vi "Calculator.vi"() -> ()   [LabVIEW 2014]
uses:
  Calc_States.ctl
panel:
  in  "stop":bool
  out "Operator_In?":bool
  out "Result":dbl
  out "Operator":string
  out "Operand_2":dbl
  out "Operand_1":dbl
  in  ".":bool caption="1 18"
  out "Numeric Indicator":dbl format="%#.13g"
  in  "=":bool caption="1 17"
  in  "%":bool caption="1 16"
  in  "Clr":bool caption="1 15"
  in  "+":bool caption="1 14"
  in  "0":bool caption="1 13"
  in  "/":bool caption="1 12"
  in  "*":bool caption="1 11"
  in  "-":bool caption="1 10"
  in  "9":bool caption="1 9"
  in  "8":bool caption="1 8"
  in  "7":bool
  in  "6":bool caption="1 6"
  in  "5":bool caption="1 5"
  in  "4":bool caption="1 4"
  in  "3":bool caption="1 3"
  in  "2":bool caption="1 2"
  in  "1":bool
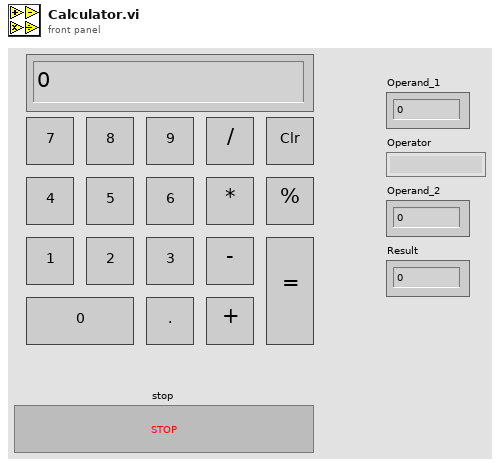
[diagram p1: front panel]
types:
  T1 = typedef "Calc_States.ctl" = cluster{"Calculator State":string, "Key Value":i16}
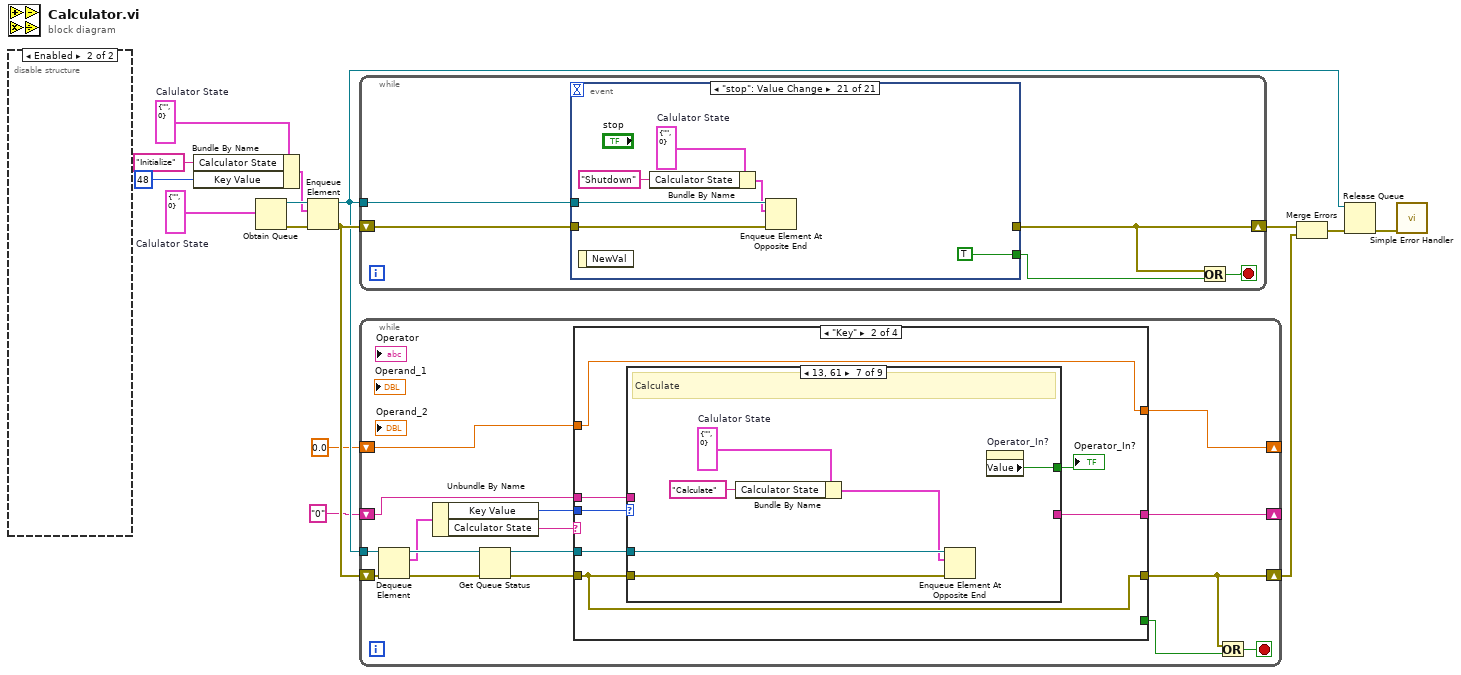
[diagram p0: block diagram]
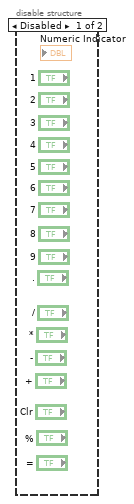
[diagram p2: hidden frame]
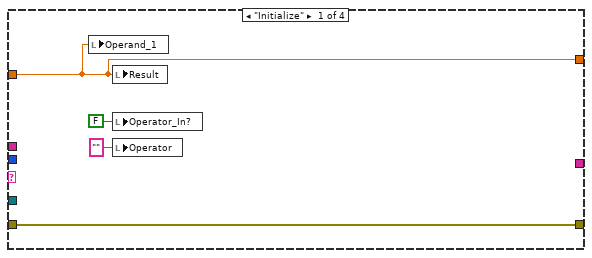
[diagram p3: hidden frame]
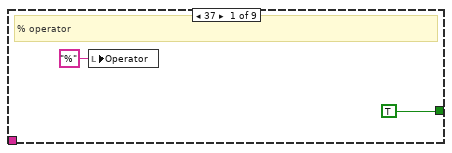
[diagram p4: hidden frame]
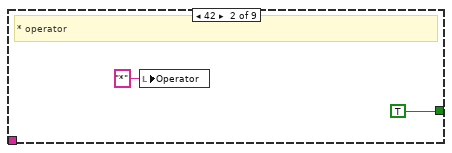
[diagram p5: hidden frame]
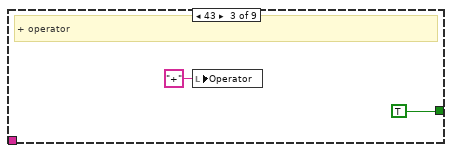
[diagram p6: hidden frame]
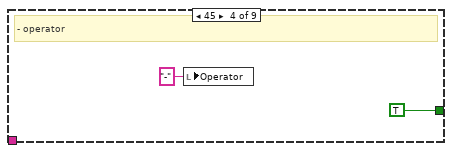
[diagram p7: hidden frame]
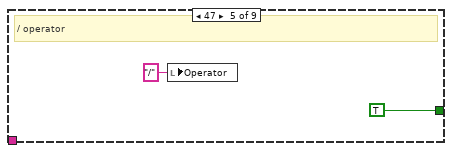
[diagram p8: hidden frame]
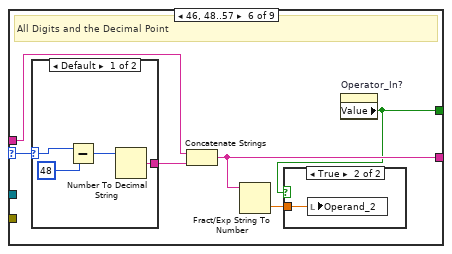
[diagram p9: hidden frame]
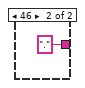
[diagram p10: hidden frame]
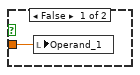
[diagram p11: hidden frame]
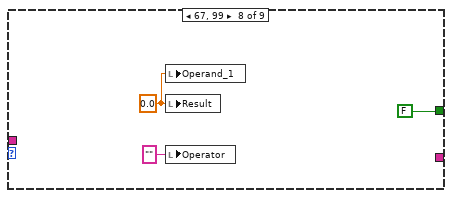
[diagram p12: hidden frame]
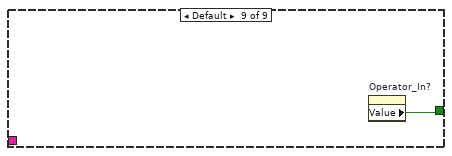
[diagram p13: hidden frame]
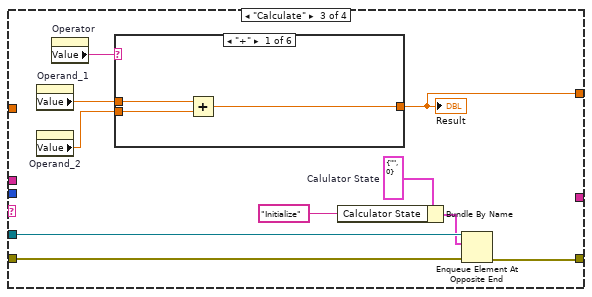
[diagram p14: hidden frame]
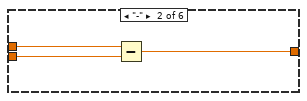
[diagram p15: hidden frame]
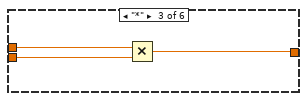
[diagram p16: hidden frame]
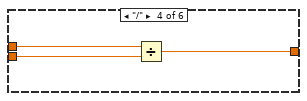
[diagram p17: hidden frame]
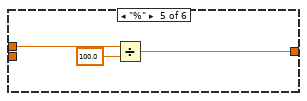
[diagram p18: hidden frame]
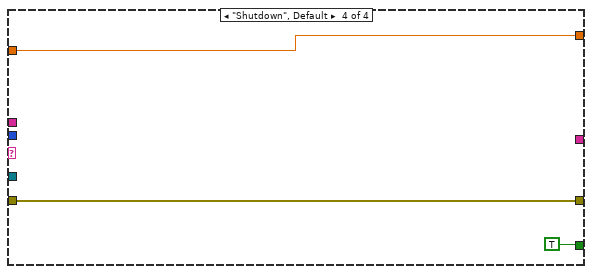
[diagram p20: hidden frame]
diagram:
  w3 = T1 {"Calculator State"="", "Key Value"=0}  # Calulator State
  w8 = T1 {"Calculator State"="", "Key Value"=0}  # Calulator State
  n1 = disable-structure shown="Enabled" {
    frame Disabled {
    }
    frame Enabled {
    }
  }
  n2 = Bundle By Name(cluster=w8, "Calculator State"="Initialize", "Key Value"=i16 48) -> (w7:T1)
  n3 = Obtain Queue(element data type=w3) -> (queue out=w14:refnum<queue>, error out=w15:errorcluster)  [unwired: 4 in, 1 out]
  n4 = Enqueue Element(queue=w14, element=w7, error in (no error)=w15) -> (queue out=w9:refnum<queue>, error out=w10:errorcluster)  [unwired: 1 in, 1 out]
  n5 = while {
    tunnel: w9 -> [w20]
    shift-right: [w17] -> w12
    shift-left: w10 -> [w19]
    stop <- w16 stop-if-true
    n6 = event shown="[20] \"stop\": Value Change" {
      selector: _ -> [_ _ _ _ _ _ _ _ _ _ _ _ _ _ _ _ _ _ _ _ _]
      dyn-events: _ -> [_ _ _ _ _ _ _ _ _ _ _ _ _ _ _ _ _ _ _ _ _]
      timeout: _ -> [_ _ _ _ _ _ _ _ _ _ _ _ _ _ _ _ _ _ _ _ _]
      tunnel: w20 -> [_ _ w27 _ _ _ _ _ _ _ _ _ _ _ _ _ _ _ _ _ w32]
      tunnel: w19 -> [_ _ w26 _ _ _ _ _ _ _ _ _ _ _ _ _ _ _ _ _ w31]
      tunnel: [_ _ w25 _ _ _ _ _ _ _ _ _ _ _ _ _ _ _ _ _ _] -> w17
      tunnel: [_ _ _ _ _ _ _ _ _ _ _ _ _ _ _ _ _ _ _ _ TRUE] -> w18
      event Timeout {
        n7 = event-data() -> ()  [unwired: 1 in, 3 out]
      }
      event "0": Value Change {
        n8 = event-data() -> ()  [unwired: 1 in, 1 out]
      }
      event Key Down {
        w24 = T1 {"Calculator State"="", "Key Value"=0}  # Calulator State
        n9 = event-data() -> ("Char"=w23:i16)  [unwired: 1 in]
        n10 = Bundle By Name(cluster=w24, "Key Value"=w23, "Calculator State"="Key") -> (w22:T1)
        n11 = Enqueue Element(queue=w27, element=w22, error in (no error)=w26) -> (error out=w25:errorcluster)  [unwired: 1 in, 2 out]
      }
      event "1": Value Change {
        n12 = event-data() -> ()  [unwired: 1 in, 6 out]
      }
      event "2": Value Change {
        n13 = event-data() -> ()  [unwired: 1 in, 6 out]
      }
      event "3": Value Change {
        n14 = event-data() -> ()  [unwired: 1 in, 6 out]
      }
      event "4": Value Change {
        n15 = event-data() -> ()  [unwired: 1 in, 6 out]
      }
      event "5": Value Change {
        n16 = event-data() -> ()  [unwired: 1 in, 6 out]
      }
      event "6": Value Change {
        n17 = event-data() -> ()  [unwired: 1 in, 6 out]
      }
      event "7": Value Change {
        n18 = event-data() -> ()  [unwired: 1 in, 6 out]
      }
      event "8": Value Change {
        n19 = event-data() -> ()  [unwired: 1 in, 6 out]
      }
      event "9": Value Change {
        n20 = event-data() -> ()  [unwired: 1 in, 6 out]
      }
      event "-": Value Change {
        n21 = event-data() -> ()  [unwired: 1 in, 6 out]
      }
      event "*": Value Change {
        n22 = event-data() -> ()  [unwired: 1 in, 6 out]
      }
      event "/": Value Change {
        n23 = event-data() -> ()  [unwired: 1 in, 6 out]
      }
      event "+": Value Change {
        n24 = event-data() -> ()  [unwired: 1 in, 6 out]
      }
      event "Clr": Value Change {
        n25 = event-data() -> ()  [unwired: 1 in, 6 out]
      }
      event "%": Value Change {
        n26 = event-data() -> ()  [unwired: 1 in, 6 out]
      }
      event "=": Value Change {
        n27 = event-data() -> ()  [unwired: 1 in, 6 out]
      }
      event ".": Value Change {
        n28 = event-data() -> ()  [unwired: 1 in, 6 out]
      }
      event "stop": Value Change {
        w29 = T1 {"Calculator State"="", "Key Value"=0}  # Calulator State
        n29 = event-data() -> ()  [unwired: 1 in, 1 out]
        n30 = Bundle By Name(cluster=w29, "Calculator State"="Shutdown") -> (w28:T1)
        n31 = Enqueue Element At Opposite End(queue=w32, element=w28, error in (no error)=w31) -> ()  [unwired: 1 in, 3 out]
      }
    }
    n32 = Or(x=w17, y=w18) -> (x .or. y?=w16:bool)
  }
  n33 = while {
    tunnel: w9 -> [w49]
    shift-right: [w38] -> w4
    shift-left: w10 -> [w48]
    shift-right: [w41] -> _
    shift-left: "0" -> [w40]
    shift-right: [w36] -> _
    shift-left: 0.0 ("Value") -> [w35]
    stop <- w34 stop-if-true
    n34 = Dequeue Element(queue=w49, error in (no error)=w48) -> (queue out=w45:refnum<queue>, element=w44:T1, error out=w47:errorcluster)  [unwired: 1 in, 1 out]
    n35 = Unbundle By Name(w44) -> ("Key Value"=w42:i16, "Calculator State"=w43:string)
    n36 = Get Queue Status(queue=w45, error in (no error)=w47) -> (queue out=w39:refnum<queue>, error out=w46:errorcluster)  [unwired: 1 in, 6 out]
    n37 = case shown="\"Key\"" w43 {
      tunnel: w46 -> [w53 w55 w100 w122]
      tunnel: [w53 w55 w99 w122] -> w38
      tunnel: w42 -> [_ w60 _ _]
      tunnel: [_ w58 _ _] -> w41
      tunnel: w40 -> [_ w57 _ _]
      tunnel: w39 -> [_ w56 w98 _]
      tunnel: w35 -> [w50 w54 _ w120]
      tunnel: [_ _ _ TRUE] -> w37
      tunnel: [w50 w54 w94 w120] -> w36
      frame "Initialize" {
        n38 = local write "Operand_1"(w50) -> ()
        n39 = local write "Result"(w50) -> ()
        n40 = local write "Operator_In?"(FALSE ("Operator_In?")) -> ()
        n41 = local write "Operator"("" ("Operator")) -> ()
      }
      frame "Key" {
        n42 = case shown="13, 61" w60 {
          selector: w60 -> [_ _ _ _ _ w72 _ _ _]
          tunnel: [TRUE TRUE TRUE TRUE TRUE w74 w89 FALSE ("Operator_In?") w93] -> w59
          tunnel: [_ _ _ _ _ w75 _ _ _] -> w58
          tunnel: w57 -> [_ _ _ _ _ w76 _ _ _]
          tunnel: w56 -> [_ _ _ _ _ _ w88 _ _]
          tunnel: w55 -> [_ _ _ _ _ _ w87 _ _]
          frame 37 {
            # "% operator"
            n43 = local write "Operator"("%" ("Operator")) -> ()
          }
          frame 42 {
            # "* operator"
            n44 = local write "Operator"("*" ("Operator")) -> ()
          }
          frame 43 {
            # "+ operator"
            n45 = local write "Operator"("+" ("Operator")) -> ()
          }
          frame 45 {
            # "- operator"
            n46 = local write "Operator"("-" ("Operator")) -> ()
          }
          frame 47 {
            # "/ operator"
            n47 = local write "Operator"("/" ("Operator")) -> ()
          }
          frame 46, 48..57 {
            # "All Digits and the Decimal Point"
            n48 = case shown="Default" w72 {
              selector: w72 -> [w79 _]
              tunnel: [w77 "."] -> w71
              frame Default {
                n49 = Subtract(x=w79, y=i16 48) -> (x-y=w78:i16)
                n50 = Number To Decimal String(number=w78) -> (decimal integer string=w77:string)  [unwired: 1 in]
              }
              frame 46 {
              }
            }
            n51 = Concatenate Strings(w76, w71) -> (w75:string)
            n52 = Fract/Exp String To Number(string=w75) -> (number=w73:dbl)  [unwired: 3 in, 1 out]
            n53 = property on="Operator_In?" class="Bool (strict)"() -> ("Value"=w74:bool)  [unwired: 2 in, 2 out]
            n54 = case shown="True" w74 {
              tunnel: w73 -> [w82 w83]
              frame False {
                n55 = local write "Operand_1"(w82) -> ()
              }
              frame True {
                n56 = local write "Operand_2"(w83) -> ()
              }
            }
          }
          frame 13, 61 {
            w85 = T1 {"Calculator State"="", "Key Value"=0}  # Calulator State
            # "Calculate"
            n57 = Bundle By Name(cluster=w85, "Calculator State"="Calculate") -> (w84:T1)
            n58 = Enqueue Element At Opposite End(queue=w88, element=w84, error in (no error)=w87) -> ()  [unwired: 1 in, 3 out]
            n59 = property on="Operator_In?" class="Bool (strict)"() -> ("Value"=w89:bool)  [unwired: 2 in, 2 out]
          }
          frame 67, 99 {
            w92 = 0.0 ("Result")
            n60 = local write "Operand_1"(w92) -> ()
            n61 = local write "Result"(w92) -> ()
            n62 = local write "Operator"("" ("Operator")) -> ()
          }
          frame Default {
            n63 = property on="Operator_In?" class="Bool (strict)"() -> ("Value"=w93:bool)  [unwired: 2 in, 2 out]
          }
        }
        "Operator_In?" <- w59
      }
      frame "Calculate" {
        w96 = T1 {"Calculator State"="", "Key Value"=0}  # Calulator State
        n64 = property on="Operand_1" class="DigNum (strict)"() -> ("Value"=w102:dbl)  [unwired: 2 in, 2 out]
        n65 = property on="Operand_2" class="DigNum (strict)"() -> ("Value"=w101:dbl)  [unwired: 2 in, 2 out]
        n66 = property on="Operator" class="Str"() -> ("Value"=w103:string)  [unwired: 2 in, 2 out]
        n67 = case shown="\"+\"" w103 {
          tunnel: w102 -> [w106 w109 w112 w115 w118 w119]
          tunnel: w101 -> [w105 w108 w111 w114 _ _]
          tunnel: [w104 w107 w110 w113 w116 w119] -> w94
          frame "+" {
            n68 = Add(x=w106, y=w105) -> (x+y=w104:dbl)
          }
          frame "-" {
            n69 = Subtract(x=w109, y=w108) -> (x-y=w107:dbl)
          }
          frame "*" {
            n70 = Multiply(x=w112, y=w111) -> (x*y=w110:dbl)
          }
          frame "/" {
            n71 = Divide(x=w115, y=w114) -> (x/y=w113:dbl)
          }
          frame "%" {
            n72 = Divide(x=w118, y=100.0) -> (x/y=w116:dbl)
          }
          frame Default {
          }
        }
        "Result" <- w94
        n73 = Bundle By Name(cluster=w96, "Calculator State"="Initialize") -> (w95:T1)
        n74 = Enqueue Element At Opposite End(queue=w98, element=w95, error in (no error)=w100) -> (error out=w99:errorcluster)  [unwired: 1 in, 2 out]
      }
      frame "Shutdown", Default {
      }
    }
    n75 = Or(x=w38, y=w37) -> (x .or. y?=w34:bool)
  }
  n76 = Merge Errors(w12, w4) -> (w13:errorcluster)
  n77 = Release Queue(queue=w9, error in (no error)=w13) -> (error out=w11:errorcluster)  [unwired: 1 in, 2 out]
  n78 = call <vilib>:"Simple Error Handler.vi"("error in (no error)"=w11) -> ()  [unwired: 4 in, 5 out]
